vi "GetButtons.vi"() -> (0 "Scale High":bool, 1 "Scale Mid":bool, 2 "Scale Low":bool, 3 "Switch":bool, 4 "Scale High 2":bool, 5 "Scale Mid 2":bool, 6 "Scale Low 2":bool, 7 "Switch 2":bool, 8 "Exchange In":bool, 9 "Exchange Out":bool, 10 "Claw Open":bool, 11 "Claw Close":bool, 12 "Rollers In":bool, 13 "Rollers Out":bool, 14 "Stow":bool, 15 "Elevator Bump Up":bool, 16 "Elevator Bump Down":bool, 17 "Wrist Out":bool, 18 "Wrist Stow":bool, 19 "Wrist Score":bool)   [LabVIEW 2018]
uses:
  <vilib>/Rock Robotics/WPI/Utilities/WPI_GetSetVariantRefNum.vi
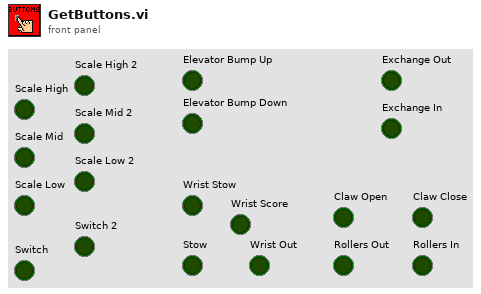
[diagram p1: front panel]
types:
  T1 = typedef "WPI_JoystickDevRef.ctl" = cluster{"Device":T2}
  T2 = typedef "WPI_JoystickDeviceEnum.ctl" = enum16{"USB 0", "USB 1", "USB 2", "USB 3", "USB 4", "USB 5"}
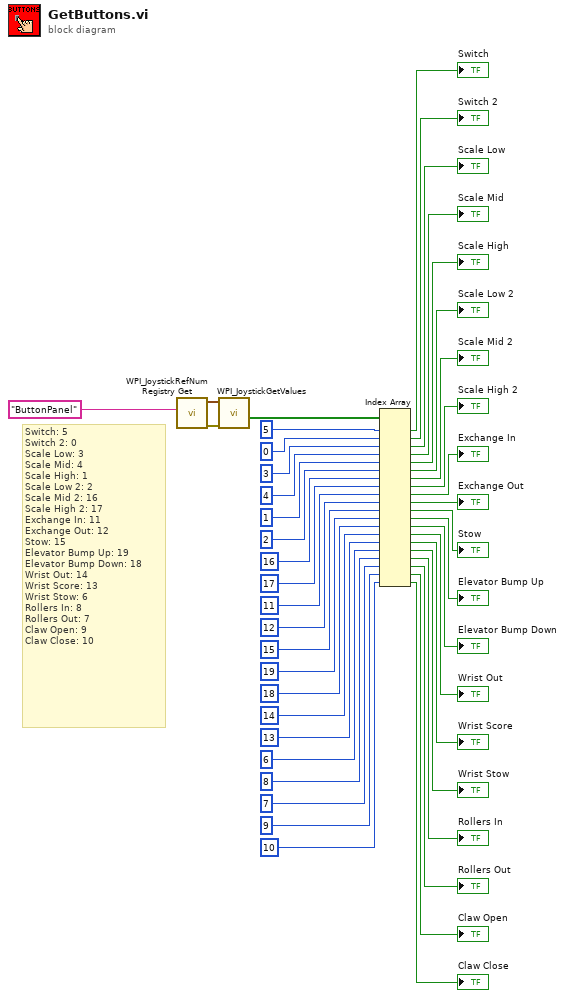
[diagram p0: block diagram]
diagram:
  # "Switch: 5\nSwitch 2: 0\nScale Low: 3\nScale Mid: 4\nScale High: 1\nScale Low 2: 2\nScale Mid 2: 16\nScale High 2: 17\nExchange In: 11\nExchange Out: 12\nStow: 15\nElevator Bump Up: 19\nElevator Bump Down: 18\nWrist Out: 14\nWrist Score: 13\nWrist Stow: 6\nRollers In: 8\nRollers Out: 7\nClaw Open: 9\nClaw Close: 10"
  n1 = call <vilib>:"WPI_JoystickRefNum Registry Get.vi"("refnum name"="ButtonPanel") -> ("error out"=w43:errorcluster, "JoystickDevRef"=w42:T1)  [unwired: 9 in]
  n2 = call <vilib>:"WPI_JoystickGetValues.vi"("error in (no error)"=w43, "JoystickDevRef"=w42) -> ("Buttons"=w41:bool[])  [unwired: 5 in, 4 out]
  n3 = Index Array(array=w41, index #1=5 ("index"), index #2=0 ("index"), index #3=3 ("index"), index #4=4 ("index"), index #5=1 ("index"), index #6=2 ("index"), index #7=16 ("index"), index #8=17 ("index"), index #9=11 ("index"), index #10=12 ("index"), index #11=15 ("index"), index #12=19 ("index"), index #13=18 ("index"), index #14=14 ("index"), index #15=13 ("index"), index #16=6 ("index"), index #17=8 ("index"), index #18=7 ("index"), index #19=9 ("index"), index #20=10 ("index")) -> (element #1=→"Switch":bool, element #2=→"Switch 2":bool, element #3=→"Scale Low":bool, element #4=→"Scale Mid":bool, element #5=→"Scale High":bool, element #6=→"Scale Low 2":bool, element #7=→"Scale Mid 2":bool, element #8=→"Scale High 2":bool, element #9=→"Exchange In":bool, element #10=→"Exchange Out":bool, element #11=→"Stow":bool, element #12=→"Elevator Bump Up":bool, element #13=→"Elevator Bump Down":bool, element #14=→"Wrist Out":bool, element #15=→"Wrist Score":bool, element #16=→"Wrist Stow":bool, element #17=→"Rollers In":bool, element #18=→"Rollers Out":bool, element #19=→"Claw Open":bool, element #20=→"Claw Close":bool)
